vi "BME_DG_Errors.vi"(8 "error in (no error)":errorcluster, 10 "source":string="Setting Delays", 11 "error":i32(ring)=503010 items=["Channel refers itself"=503001, "Deadloop"=503002, "Negative Delay"=503003]) -> (0 "error out":errorcluster)   [LabVIEW 2009]
uses:
  <vilib>/Utility/error.llb/DialogType.ctl
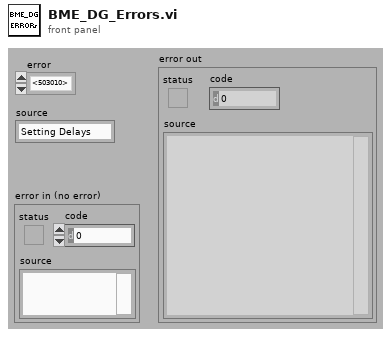
[diagram p1: front panel]
types:
  T1 = typedef "DialogType.ctl" = u16
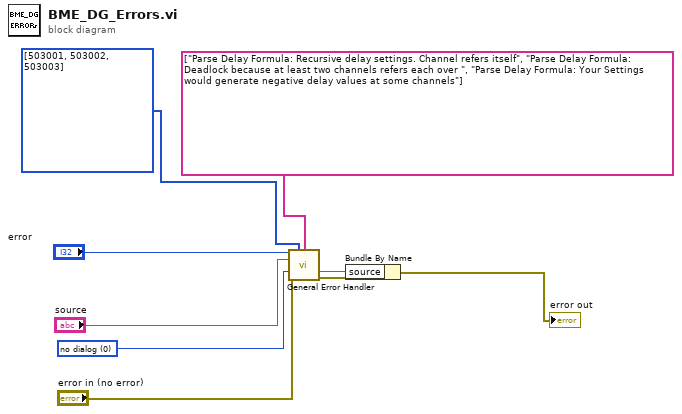
[diagram p0: block diagram]
diagram:
  w5 = T1 0 items=["no dialog", "OK message", "continue or stop message", "OK message + warnings", "continue/stop + warnings"] ("type of dialog (OK msg:1)")
  n1 = call <vilib>:"General Error Handler.vi"("[error code] (0)"="error", "[user-defined codes]"=i32[] [503001, 503002, 503003], "[user-defined descriptions]"=string[] ["Parse Delay Formula: Recursive delay settings. Channel refers itself", "Parse Delay Formula: Deadlock because at least two channels refers each over ", "Parse Delay Formula: Your Settings would generate negative delay values at some channels"], "[error source] (\" \")"="source", "type of dialog (OK msg:1)"=w5, "error in (no error)"="error in (no error)") -> ("message"=w1:string, "error out"=w3:errorcluster)  [unwired: 5 in, 3 out]
  n2 = Bundle By Name(cluster=w3, "source"=w1) -> (→"error out":errorcluster)
